vi "OP300ZP_SEALING.vi"(8 "ERRIN":errorcluster caption="entrée d'erreur (pas d'erreur)") -> (0 "ERROUT":errorcluster caption="sortie d'erreur", 2 "SEALING_VALUE":dbl, 3 "IsOK?":bool)   [LabVIEW 2020]
uses:
  <instrlib>/HIOKI BT356X Series/HIOKI BT356X Series.lvlib
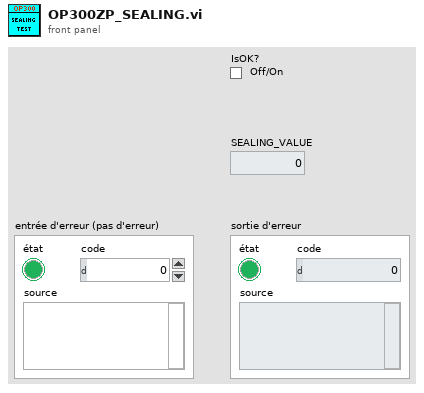
[diagram p1: front panel]
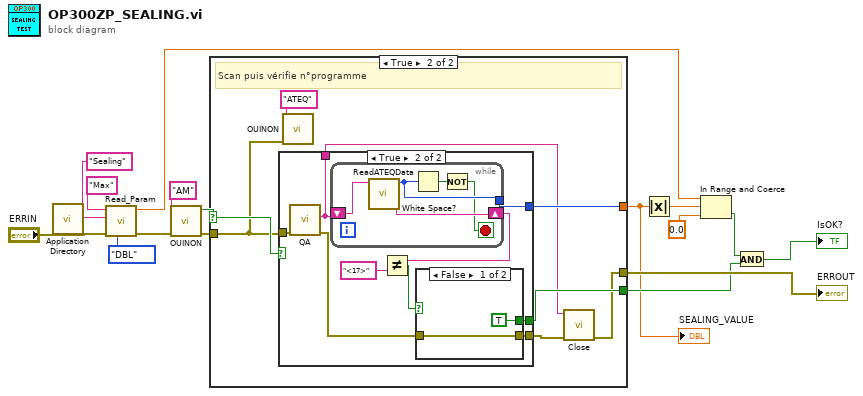
[diagram p0: block diagram]
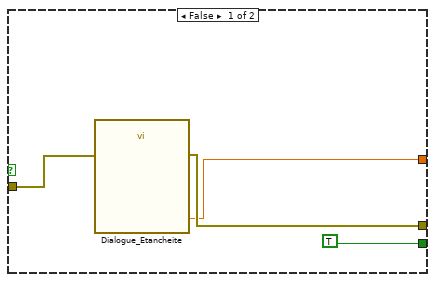
[diagram p2: hidden frame]
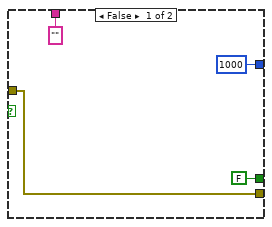
[diagram p3: hidden frame]
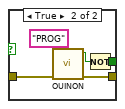
[diagram p4: hidden frame]
diagram:
  n1 = call <vilib>:"Application Directory.vi"() -> ()  [unwired: 1 out]
  n2 = call <userlib>:"Read_Param.vi"("Énum"=enum16{"STR", "DBL", "U32"}."DBL", "errin"="ERRIN", "section"="Sealing", "key"="Max") -> ("error out"=w6:errorcluster, "dbl"=w10:dbl)  [unwired: 3 in, 3 out]
  n3 = call <userlib>:"OUINON.vi"("errin"=w6, "image"="AM" ("IN")) -> ("error out"=w4:errorcluster, "OUI/NON"=w5:bool)  [unwired: 8 in]
  n4 = case shown="True" w5 {
    selector: w5 -> [_ w25]
    tunnel: [w19 w28] -> w2
    tunnel: [w20 w22] -> w15
    tunnel: [TRUE w27] -> w8
    tunnel: w4 -> [w17 w24]
    frame False {
      n5 = call "Dialogue_Etancheite.vi"("error in (no error)"=w17) -> ("Valeur d'étanchéité"=w19:dbl, "error out"=w20:errorcluster)  [unwired: 16 in, 1 out]
    }
    frame True {
      # "Scan puis vérifie n°programme"
      n6 = case shown="True" w25 {
        tunnel: [1000 ("Valeur") w41] -> w28
        tunnel: [w32 w39] -> w23
        tunnel: [FALSE w38] -> w27
        tunnel: w24 -> [w32 w34]
        tunnel: ["" ("DATAOUT") w33] -> w21
        frame False {
        }
        frame True {
          n7 = call "QA.vi"("ERRIN"=w34) -> ("ERROUT"=w40:errorcluster, "DATAOUT"=w33:string)  [unwired: 9 in]
          n8 = while {
            tunnel: [w46] -> w41
            shift-right: [w44] -> w37
            shift-left: w33 -> [w45]
            stop <- w42 stop-if-true
            n9 = call "ReadATEQData.vi"("Chaîne"=w45) -> ("Prg number"=w44:string, "Valeur"=w46:i32)  [unwired: 7 in, 2 out]
            n10 = White Space?(1:w46) -> (0:w43:bool)
            n11 = Not(x=w43) -> (.not. x?=w42:bool)
          }
          n12 = Not Equal?(x=w37, y="<17>") -> (x != y?=w35:bool)
          n13 = case shown="False" w35 {
            tunnel: w40 -> [w47 w52]
            tunnel: [w47 w51] -> w39
            tunnel: [TRUE w49] -> w38
            frame False {
            }
            frame True {
              n14 = call <userlib>:"OUINON.vi"("errin"=w52, "image"="PROG" ("IN")) -> ("error out"=w51:errorcluster, "OUI/NON"=w50:bool)  [unwired: 8 in]
              n15 = Not(x=w50) -> (.not. x?=w49:bool)
            }
          }
        }
      }
      n16 = call <userlib>:"OUINON.vi"("errin"=w24, "image"="ATEQ" ("IN")) -> ()  [unwired: 8 in, 2 out]
      n17 = call <instrlib>:"Close.vi"("error in (no error)"=w23, "VISA resource name"=w21) -> ("error out"=w22:errorcluster)  [unwired: 9 in]
    }
  }
  "SEALING_VALUE" <- w2
  "ERROUT" <- w15
  n18 = Absolute Value(x=w2) -> (abs(x)=w1:dbl)
  n19 = In Range and Coerce ("Dans la gamme")(upper limit=w10, x=w1, lower limit=0.0 ("limite inférieure")) -> (In Range?=w9:bool)  [unwired: 1 out]
  n20 = And(x=w9, y=w8) -> (x .and. y?=→"IsOK?":bool)
